vi "BinanceAPI_EXMPLE.vi"() -> ()   [LabVIEW 2022 SP3, in "BinanceAPI_.lvclass"]
doc: "Simple example. Any API key is not required.\n\nBut API keys is nessesery for other functions.\n\nLOG INTO BINANCE AND IN \"API MANAGMENT\" CREATE API KEYS\n\nMARK:\n - FUTURES CONTRACTS\n - ENABLE READ\n - NO IP FILTER (LATER YOU CAN SET YOUR OWN)\n - ENABLE SPOT AND MARGIN\n\nATTENTION!!! SAVE YOUR SECRED KEY BECOUSE YOU SEE IT LAST TIME."
uses:
  src/BinanceAPI_.lvclass
  src/GET/All_Get_Functions/_API_BINANCE_GET_Price.vi
panel:
  out "value":cluster{"price":string, "symbol":string}
  out "Body":string
  in  "stop":bool
  out "Waveform Chart":dbl(graph)
  in  "Secred API":string
  in  "API KEY":string
  in  "symbol (e.g. BTCUSDT)":string="BTCUSDT"
  out "error out":errorcluster
  in  "error in (no error)":errorcluster
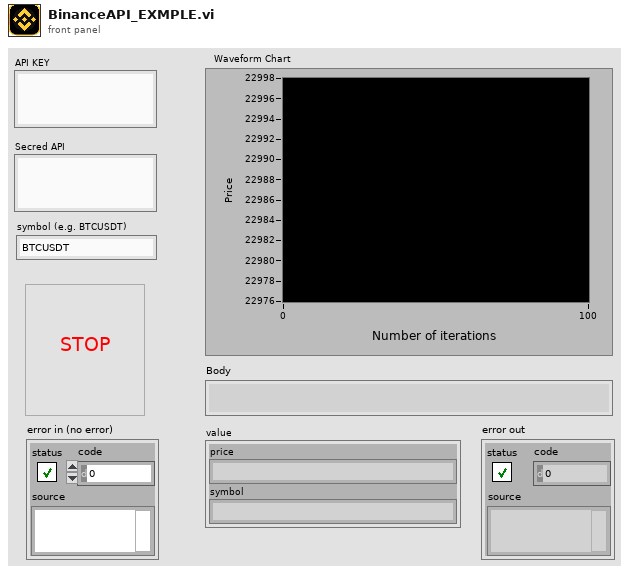
[diagram p1: front panel]
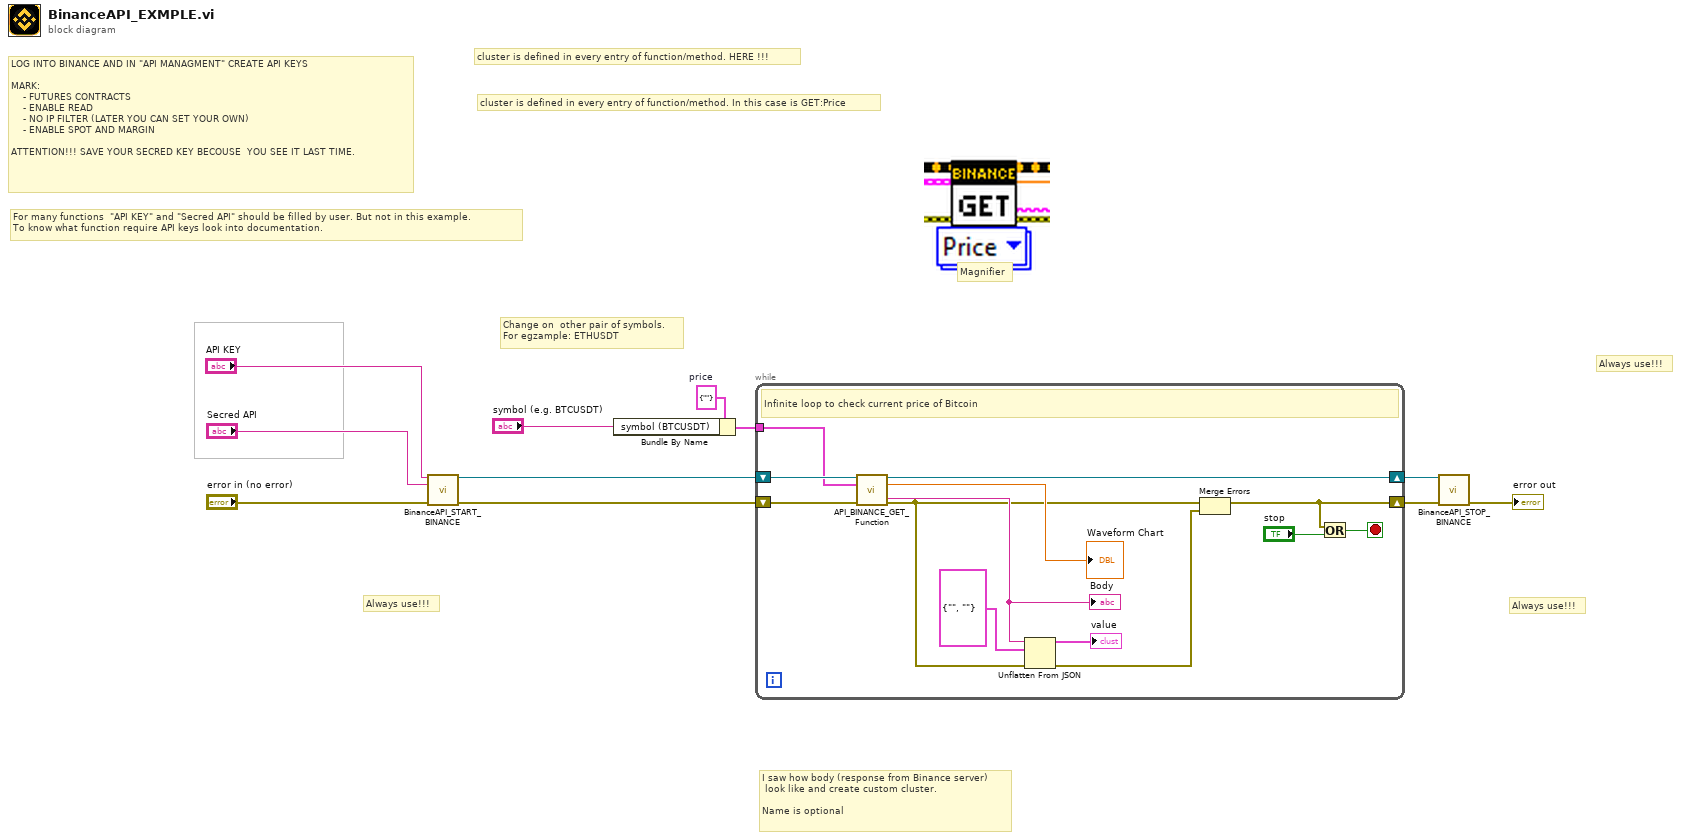
[diagram p0: block diagram]
diagram:
  w3 = cluster{"symbol (BTCUSDT)":string} {"symbol (BTCUSDT)"=""}  # price
  # "Change on  other pair of symbols.\nFor egzample: ETHUSDT"
  # "LOG INTO BINANCE AND IN \"API MANAGMENT\" CREATE API KEYS\n\nMARK:\n    - FUTURES CONTRACTS\n    - ENABLE READ\n    - NO IP FILTER (LATER YOU CAN SET YOUR OWN)\n    - ENABLE SPOT AND MARGIN\n\nATTENTION!!! SAVE YOUR SECRED KEY BECOUSE  YOU SEE IT LAST TIME."
  # "cluster is defined in every entry of function/method. HERE !!!"
  # "cluster is defined in every entry of function/method. In this case is GET:Price"
  # "Magnifier"
  # "Always use!!!"
  # "Always use!!!"
  # "Always use!!!"
  # "I saw how body (response from Binance server)\n look like and create custom cluster.\n\nName is optional"
  # "For many functions  \"API KEY\" and \"Secred API\" should be filled by user. But not in this example.\nTo know what function require API keys look into documentation."
  n1 = call "BinanceAPI_START_BINANCE.vi"("API KEY"="API KEY", "Secred API"="Secred API", "error in (no error)"="error in (no error)") -> ("BinanceAPI"=w7:refnum<class "BinanceAPI_.lvclass">, "error out"=w6:errorcluster)  [unwired: 10 in, 1 out]
  n2 = Bundle By Name(cluster=w3, "symbol (BTCUSDT)"="symbol (e.g. BTCUSDT)") -> (w1:cluster{"symbol (BTCUSDT)":string})
  n3 = while {
    tunnel: w1 -> [w21]
    shift-right: [w22] -> w5
    shift-left: w7 -> [w24]
    shift-right: [w14] -> w4
    shift-left: w6 -> [w23]
    stop <- w12 stop-if-true
    # "Infinite loop to check current price of Bitcoin"
    n4 = call-poly "API_BINANCE_GET_Function.vi"("BinanceAPI in"=w24, "price"=w21, "error in (no error)"=w23) -> ("BinanceAPI out"=w22:refnum<class "BinanceAPI_.lvclass">, "lastPrice"=→"Waveform Chart":dbl, "Body"=w19:string, "error out"=w15:errorcluster)  [unwired: 9 in]
    "Body" <- w19
    n5 = Unflatten From JSON(JSON string=w19, type and defaults=cluster{"price":string, "symbol":string} {"price"="", "symbol"=""} ("Name is optional"), error in (no error)=w15) -> (value=→"value":cluster{"price":string, "symbol":string}, error out=w16:errorcluster)  [unwired: 4 in]
    n6 = Merge Errors(w15, w16) -> (w14:errorcluster)
    n7 = Or(x=w14, y="stop") -> (x .or. y?=w12:bool)
  }
  n8 = call "BinanceAPI_STOP_BINANCE.vi"("BinanceAPI_.lvclass"=w5, "error in (no error)"=w4) -> ("error out"=→"error out":errorcluster)  [unwired: 13 in]
